vi "Add Digital Pattern - Multi FPGA.vi"(8 "error in (no error)":errorcluster, 10 "Page Data in":T1 {"Node Ptr" format="%.0x"}, 11 "State queue in":string[](array[string])) -> (0 "error out":errorcluster, 2 "Page Data out":T1 {"Node Ptr" format="%.0x"}, 3 "State queue out":string[](array[string]))   [LabVIEW 2015, in "Engine Simulation Toolkit System Explorer.lvlib"]
uses:
  Engine Simulation Toolkit System Explorer.lvlib
  Digital Patterns Page Data.ctl
  <vilib>/NI Veristand/Custom Device API/Custom Device Item Ref.ctl
  Digital Pattern.ctl
  Digital Pattern Base.ctl
  Digital Pattern Remove Edge.ctl
  Digital Pattern Add Pulse.ctl
  <vilib>/NI Veristand/Custom Device API/Custom Device Channel Type.ctl
  Shared/Constants and GUIDs.vi
  Shared/Properties.vi
  <vilib>/NI Veristand/Custom Device API/Set Item Property (String).vi
  <vilib>/NI Veristand/Custom Device API/Custom Device API.lvlib
  Shared/Engine Simulation Toolkit Shared.lvlib
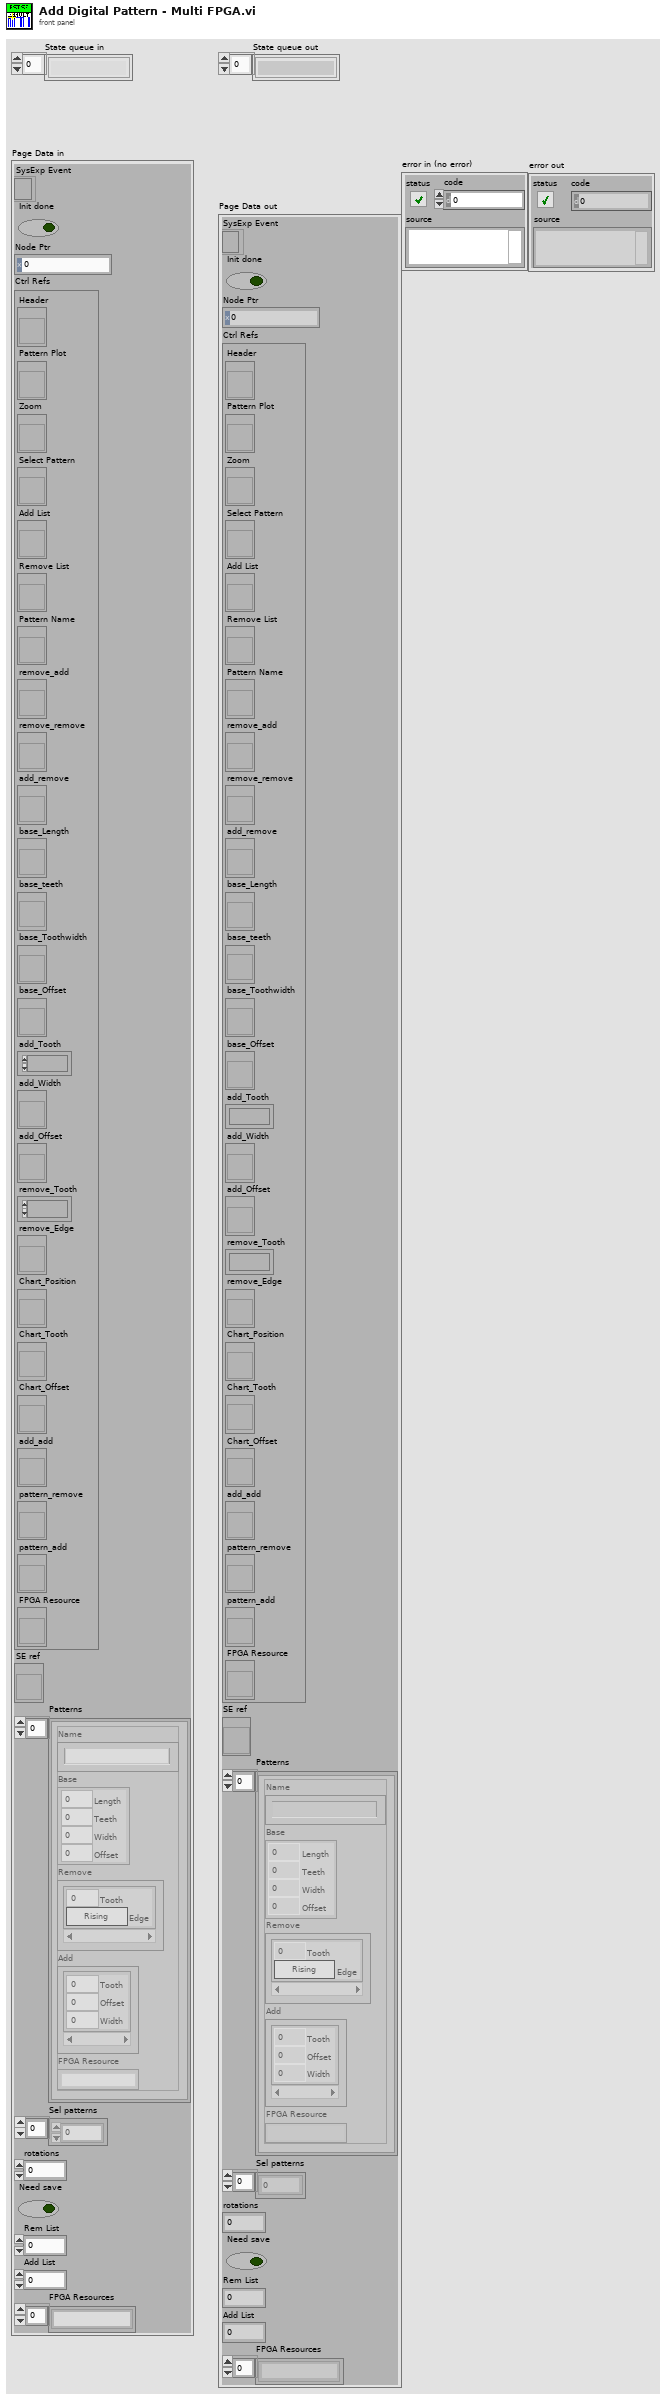
[diagram p1: front panel]
types:
  T1 = typedef "Engine Simulation Toolkit System Explorer.lvlib/Digital Patterns Page Data.ctl" = cluster{"SysExp Event":refnum<event-registration>, "Init done":bool, "Node Ptr":T2, "Ctrl Refs":cluster{"Header":refnum<vi>, "Pattern Plot":refnum<vi>, "Zoom":refnum<vi>, "Select Pattern":refnum<vi>, "Add List":refnum<vi>, "Remove List":refnum<vi>, "Pattern Name":refnum<vi>, "remove_add":refnum<vi>, "remove_remove":refnum<vi>, "add_remove":refnum<vi>, "base_Length":refnum<vi>, "base_teeth":refnum<vi>, "base_Toothwidth":refnum<vi>, "base_Offset":refnum<vi>, "add_Tooth":refnum<vi>, "add_Width":refnum<vi>, "add_Offset":refnum<vi>, "remove_Tooth":refnum<vi>, "remove_Edge":refnum<vi>, "Chart_Position":refnum<vi>, "Chart_Tooth":refnum<vi>, "Chart_Offset":refnum<vi>, "add_add":refnum<vi>, "pattern_remove":refnum<vi>, "pattern_add":refnum<vi>, "FPGA Resource":refnum<vi>}, "SE ref":refnum<vi>, "Patterns":T3[], "Sel patterns":i32[], "rotations":u16, "Need save":bool, "Rem List":i32, "Add List":i32, "FPGA Resources":string[]}
  T2 = typedef "Custom Device API.lvlib/Custom Device Item Ref.ctl" = u64
  T3 = typedef "Engine Simulation Toolkit System Explorer.lvlib/Digital Pattern.ctl" = cluster{"Name":string, "Base":T4, "Remove":T5[], "Add":T6[], "FPGA Resource":string}
  T4 = typedef "Engine Simulation Toolkit System Explorer.lvlib/Digital Pattern Base.ctl" = cluster{"Length":dbl, "Teeth":u16, "Width":dbl, "Offset":dbl}
  T5 = typedef "Engine Simulation Toolkit System Explorer.lvlib/Digital Pattern Remove Edge.ctl" = cluster{"Tooth":u16, "Edge":bool}
  T6 = typedef "Engine Simulation Toolkit System Explorer.lvlib/Digital Pattern Add Pulse.ctl" = cluster{"Tooth":u16, "Offset":dbl, "Width":dbl}
  T7 = typedef "Custom Device API.lvlib/Custom Device Channel Type.ctl" = enum16{"Input", "Output"}
  T8 = typedef "Engine Simulation Toolkit Shared.lvlib/Bitfile EST Version.ctl" = enum16{"1.0", "1.1", "1.2", "1.3"}
  T9 = typedef "Engine Simulation Toolkit Shared.lvlib/Channel.ctl" = cluster{"Name":string, "Units":string, "Default":dbl, "Description":string, "Scalable":bool}
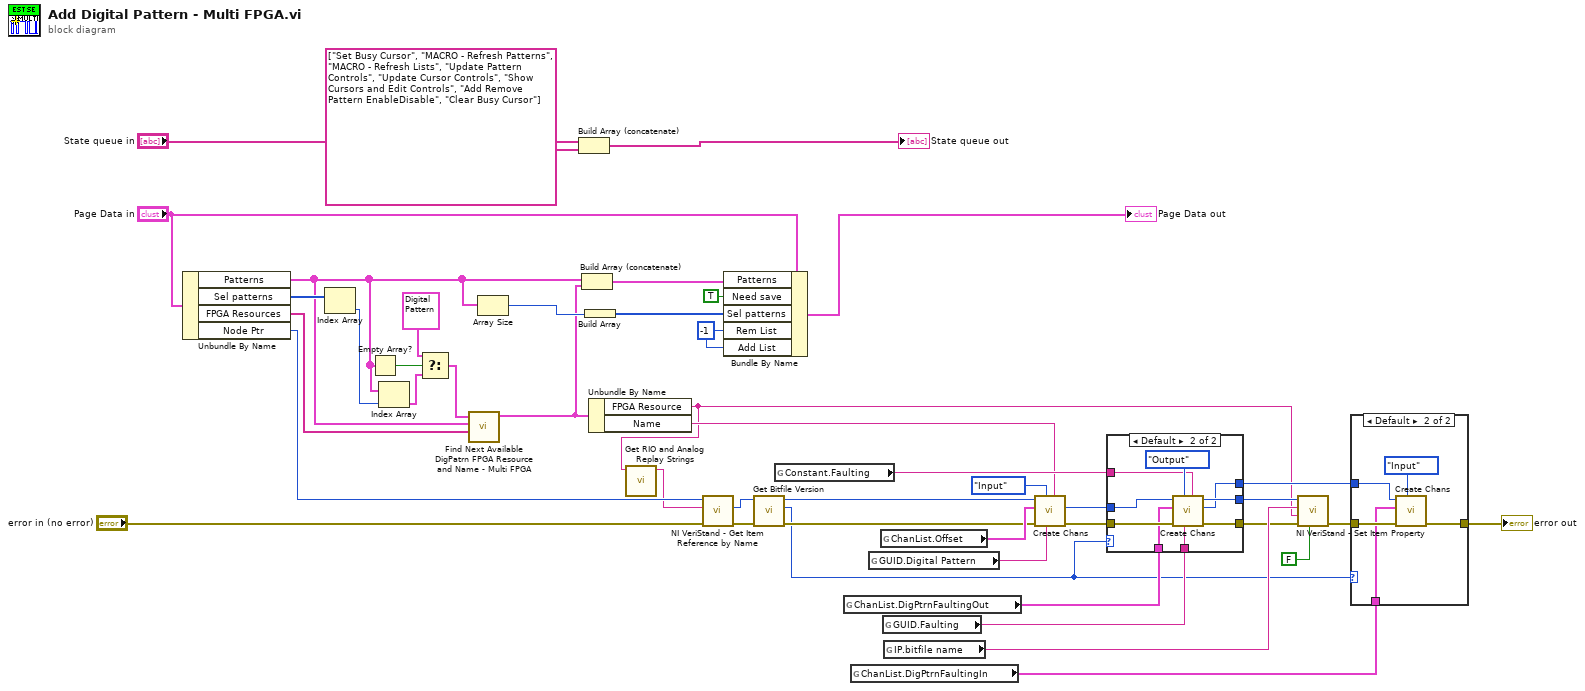
[diagram p0: block diagram]
diagram:
  w44 = -1 ("Rem List")
  n1 = Unbundle By Name("Page Data in") -> ("Patterns"=w30:T3[], "Sel patterns"=w39:i32[], "FPGA Resources"=w31:string[], "Node Ptr"=w4:T2)
  n2 = Index Array(array=w39) -> (element=w41:i32)  [unwired: 1 in]
  n3 = Empty Array?(array=w30) -> (empty?=w28:bool)
  n4 = Index Array(array=w30, index=w41) -> (element=w38:T3)
  n5 = Select(t=T3 {"Name"="New Pattern", "Base"={"Length"=360.0, "Teeth"=60, "Width"=1.0, "Offset"=-0.5}, "Remove"=[{"Tooth"=58, "Edge"=FALSE}, {"Tooth"=59, "Edge"=FALSE}], "Add"=[], "FPGA Resource"=""} ("s? t:f"), s=w28, f=w38) -> (s? t:f=w29:T3)
  n6 = call "Find Next Available DigPatrn FPGA Resource and Name - Multi FPGA.vi"("FPGA Resources"=w31, "Patterns"=w30, "New Pattern in"=w29) -> ("New Pattern out"=w27:T3)  [unwired: 8 in]
  n7 = Array Size(array=w30) -> (size(s)=w45:i32)
  n8 = Build Array (concatenate)("State queue in", string[] ["Set Busy Cursor", "MACRO - Refresh Patterns", "MACRO - Refresh Lists", "Update Pattern Controls", "Update Cursor Controls", "Show Cursors and Edit Controls", "Add Remove Pattern EnableDisable", "Clear Busy Cursor"]) -> (→"State queue out":string[])
  n9 = Build Array (concatenate)(w30, w27) -> (w40:T3[])
  n10 = Build Array(w45) -> (w42:i32[])
  n11 = Unbundle By Name(w27) -> ("FPGA Resource"=w1:string, "Name"=w2:string)
  n12 = call "Get RIO and Analog Replay Strings.vi"("rio/analog replay"=w1) -> ("rio"=w3:string)  [unwired: 9 in, 1 out]
  n13 = call <vilib>:"NI VeriStand - Get Item Reference by Name.vi"("error in (no error)"="error in (no error)", "Item Name"=w3, "Parent Ref in"=w4) -> ("error out"=w7:errorcluster, "Item Ref"=w6:T2)  [unwired: 5 in, 2 out]
  n14 = Bundle By Name(cluster="Page Data in", "Patterns"=w40, "Need save"=TRUE, "Sel patterns"=w42, "Rem List"=w44, "Add List"=w44) -> (→"Page Data out":T1)
  n15 = call "Get Bitfile Version.vi"("error in (no error)"=w7, "Item Ref in"=w6) -> ("error out"=w11:errorcluster, "EST version enum"=w9:T8, "Item Ref out"=w10:T2)  [unwired: 6 in, 1 out]
  n16 = global read "Constants and GUIDs.vi" "Constant.Faulting"() -> (w8:string)
  n17 = global read "Constants and GUIDs.vi" "ChanList.DigPtrnFaultingOut"() -> (w17:T9[])
  n18 = global read "Constants and GUIDs.vi" "ChanList.DigPtrnFaultingIn"() -> (w14:T9[])
  n19 = global read "Constants and GUIDs.vi" "GUID.Digital Pattern"() -> (w24:string)
  n20 = global read "Constants and GUIDs.vi" "ChanList.Offset"() -> (w25:T9[])
  n21 = global read "Constants and GUIDs.vi" "GUID.Faulting"() -> (w12:string)
  n22 = global read "Properties.vi" "IP.bitfile name"() -> (w22:string)
  n23 = call "Create Chans.vi"("New Section Name (none)"=w2, "new section GUID (\"\":del prot)"=w24, "Type"=Custom_Device_Channel_Type."Input", "error in (no error)"=w11, "Channels"=w25, "Section Ptr"=w10) -> ("error out"=w23:errorcluster, "new section ref"=w19:T2)  [unwired: 2 in, 2 out]
  n24 = case shown="Default" w9 {
    tunnel: w23 -> [w46 w56]
    tunnel: [w46 w55] -> w20
    tunnel: w19 -> [w47 w54]
    tunnel: [w47 w53] -> w18
    tunnel: w17 -> [_ w52]
    tunnel: [_ w50] -> w15
    tunnel: w12 -> [_ w49]
    tunnel: w8 -> [_ w48]
    frame "1.0".."1.2" {
    }
    frame Default {
      n25 = call "Create Chans.vi"("New Section Name (none)"=w48, "new section GUID (\"\":del prot)"=w49, "Type"=Custom_Device_Channel_Type."Output", "error in (no error)"=w56, "Channels"=w52, "Section Ptr"=w54) -> ("error out"=w55:errorcluster, "new section ref"=w50:T2, "Section Ptr dup"=w53:T2)  [unwired: 2 in, 1 out]
    }
  }
  n26 = call-poly <vilib>:"NI VeriStand - Set Item Property.vi"("Binary String (T)"=FALSE, "error in (no error)"=w20, "Value"=w1, "Property Name"=w22, "Item Ref in"=w18) -> ("error out"=w16:errorcluster)  [unwired: 4 in, 2 out]
  n27 = case shown="Default" w9 {
    tunnel: w16 -> [w57 w62]
    tunnel: w15 -> [_ w61]
    tunnel: w14 -> [_ w60]
    tunnel: [w57 w58] -> w13
    frame "1.0".."1.2" {
    }
    frame Default {
      n28 = call "Create Chans.vi"("Type"=Custom_Device_Channel_Type."Input", "error in (no error)"=w62, "Channels"=w60, "Section Ptr"=w61) -> ("error out"=w58:errorcluster)  [unwired: 4 in, 3 out]
    }
  }
  "error out" <- w13
